vi "Write TCPClient.vi"(8 "error in (no error)":errorcluster, 10 "TCPClient.lvclass":refnum<class "TCPClient.lvclass">, 11 "AlCS in":refnum<class "AlCS.lvclass">) -> (0 "error out":errorcluster, 3 "AlCS out":refnum<class "AlCS.lvclass">)   [LabVIEW 2016, in "AlCS.lvclass"]
uses:
  AlCS.lvclass
  ts_labview_tcp/TCPClient/TCPClient.lvclass
  AlCS.lvclass/AlCS.ctl
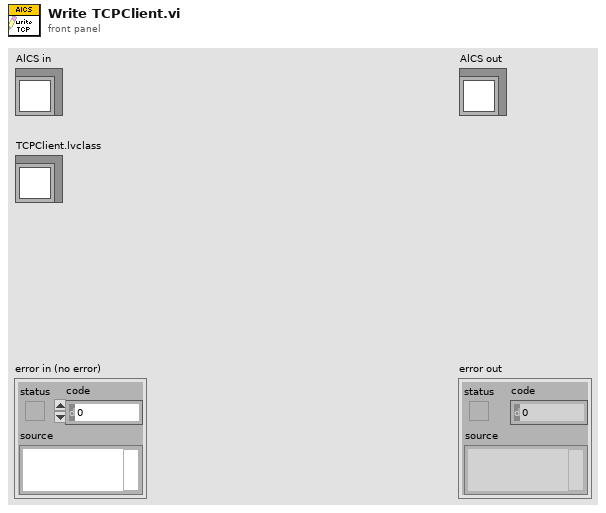
[diagram p1: front panel]
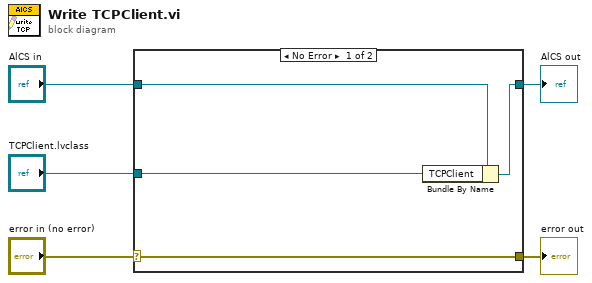
[diagram p0: block diagram]
diagram:
  n1 = case shown="No Error" "error in (no error)" {
    selector: "error in (no error)" -> [w9 w10]
    tunnel: [w9 w10] -> w4
    tunnel: [w7 w11] -> w2
    tunnel: "AlCS in" -> [w8 w11]
    tunnel: "TCPClient.lvclass" -> [w6 _]
    frame No Error {
      n2 = Bundle By Name(cluster=w8, "TCPClient"=w6) -> (w7:refnum<class "AlCS.lvclass">)
    }
    frame Error {
    }
  }
  "error out" <- w4
  "AlCS out" <- w2
